vi "C2F.vi"(10 "TempC":dbl) -> (2 "TempF":dbl)   [LabVIEW 2019]
doc: "This function calculates the Temperature in Celcius to Temperature in Farhenheit\nTempC is Input (It should be in C)\nTempF is output (It will be in F)"
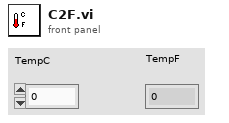
[diagram p1: front panel]
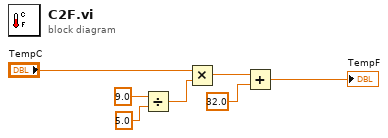
[diagram p0: block diagram]
diagram:
  n1 = Divide(x=9.0, y=5.0 ("x")) -> (x/y=w1:dbl)
  n2 = Multiply(x="TempC", y=w1) -> (x*y=w4:dbl)
  n3 = Add(x=w4, y=32.0) -> (x+y=→"TempF":dbl)
